vi "Stop lettura res.vi"() -> ()   [LabVIEW 2019]
panel:
  out "LETTURA RESISTOMAT":dbl
  out "MISURA RESISTOMAT PRONTA":bool
  out "STOP LETTURA RES":bool
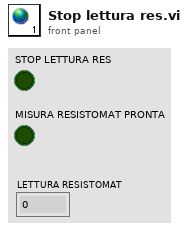
[diagram p1: front panel]
diagram:
